vi "LevMar - xx.vi"(1 "Target function in":refnum<vi>, 2 "Coefficients":dbl[](array[numeric]) format="%0.2f", 3 "Y":dbl[](array[numeric]) format="%0.2f", 4 "error":i32 caption="erreur", 8 "Standard Deviation":dbl[](array[numeric]) caption="Écart-type" format="%0.2f") -> (5 "Target function out":refnum<vi>, 7 "chiSqr":dbl caption="khiCarré" format="%0.2f")   [LabVIEW 2009]
panel:
  # "Lev-Mar\n XX"
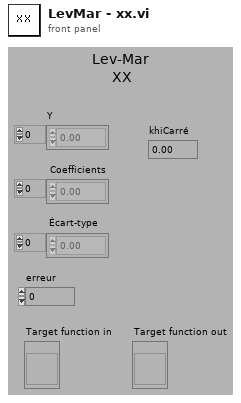
[diagram p1: front panel]
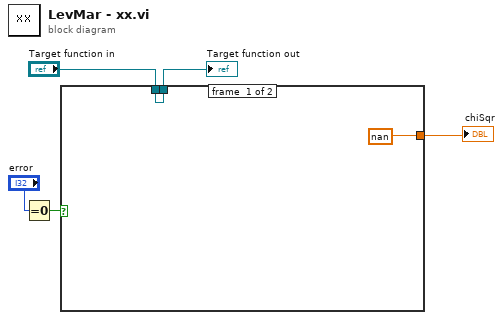
[diagram p0: block diagram]
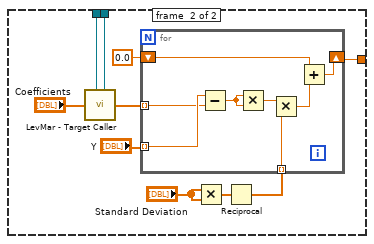
[diagram p2: hidden frame]
diagram:
  n1 = Equal To 0?(x="error") -> (x = 0?=w4:bool)
  n2 = case shown="True" w4 {
    tunnel: [nan w17] -> w3
    tunnel: "Target function in" -> [w6 w9]
    tunnel: [w6 w8] -> w1
    frame #0 {
    }
    frame #1 {
      n3 = call "LevMar - Target Caller.vi"("A"="Coefficients", "Target Function in"=w9) -> ("Target Function out"=w8:refnum<vi>, "F"=w10:dbl[])
      n4 = Multiply(x="Standard Deviation", y="Standard Deviation") -> (x*y=w13:dbl[])
      n5 = Reciprocal(x=w13) -> (1/x=w12:dbl[])
      n6 = for {
        shift-right: [w25] -> w17
        shift-left: 0.0 -> [w19]
        tunnel: "Y" -> [w24] mode=indexing
        tunnel: w12 -> [w21] mode=indexing
        tunnel: w10 -> [w20] mode=indexing
        n7 = Subtract(x=w24, y=w20) -> (x-y=w23:dbl)
        n8 = Multiply(x=w23, y=w23) -> (x*y=w22:dbl)
        n9 = Multiply(x=w22, y=w21) -> (x*y=w18:dbl)
        n10 = Add(x=w19, y=w18) -> (x+y=w25:dbl)
      }
    }
  }
  "chiSqr" <- w3
  "Target function out" <- w1
